vi "6-2_LED VI Curve.vi"() -> ()   [LabVIEW 2014]
doc: "This example demonstrates how to read N channels of analog input from a LINX device.\n------------------------------------\nAuther: Koji Ohashi\nCopyright (c) 2020 Japan LabVIEW Users Group, Volunteer members.\nThis VI is released under the MIT License.\nhttp://opensource.org/licenses/mit-license.php\n------------------------------------"
uses:
  <vilib>/MakerHub/LINX/LMH-LINX.lvlib
  <vilib>/MakerHub/LINX/Public/Peripherals/Analog/Analog Read N Chans.vi
  <vilib>/MakerHub/LINX/Public/Utilities/Open Serial.vi
panel:
  in  "Add Data":bool
  in  "regression analysis":bool
  in  "Resistor (ƒ¶)":dbl=100.0 format="%#_13g"
  out "LED VI characteristics":cluster{dbl[], dbl[]}[](graph)
  in  "AI Channel(s)":u8[](array[numeric])=[0, 1, 2]
  in  "Stop Button":bool
  out "Analog Data":T1(graph)
  in  "Serial Port":refnum<visa-resource-name>
  # "LINX Device Settings"
  # "Model formula used for regression analysis"
  # "n: Ideal diode factor\nI0: Reverse saturation current\ne: Napier number\nr: Internal resistance"
  # "e: elementary charge\nk: Boltzmann constant\nT: Absolute temperature"
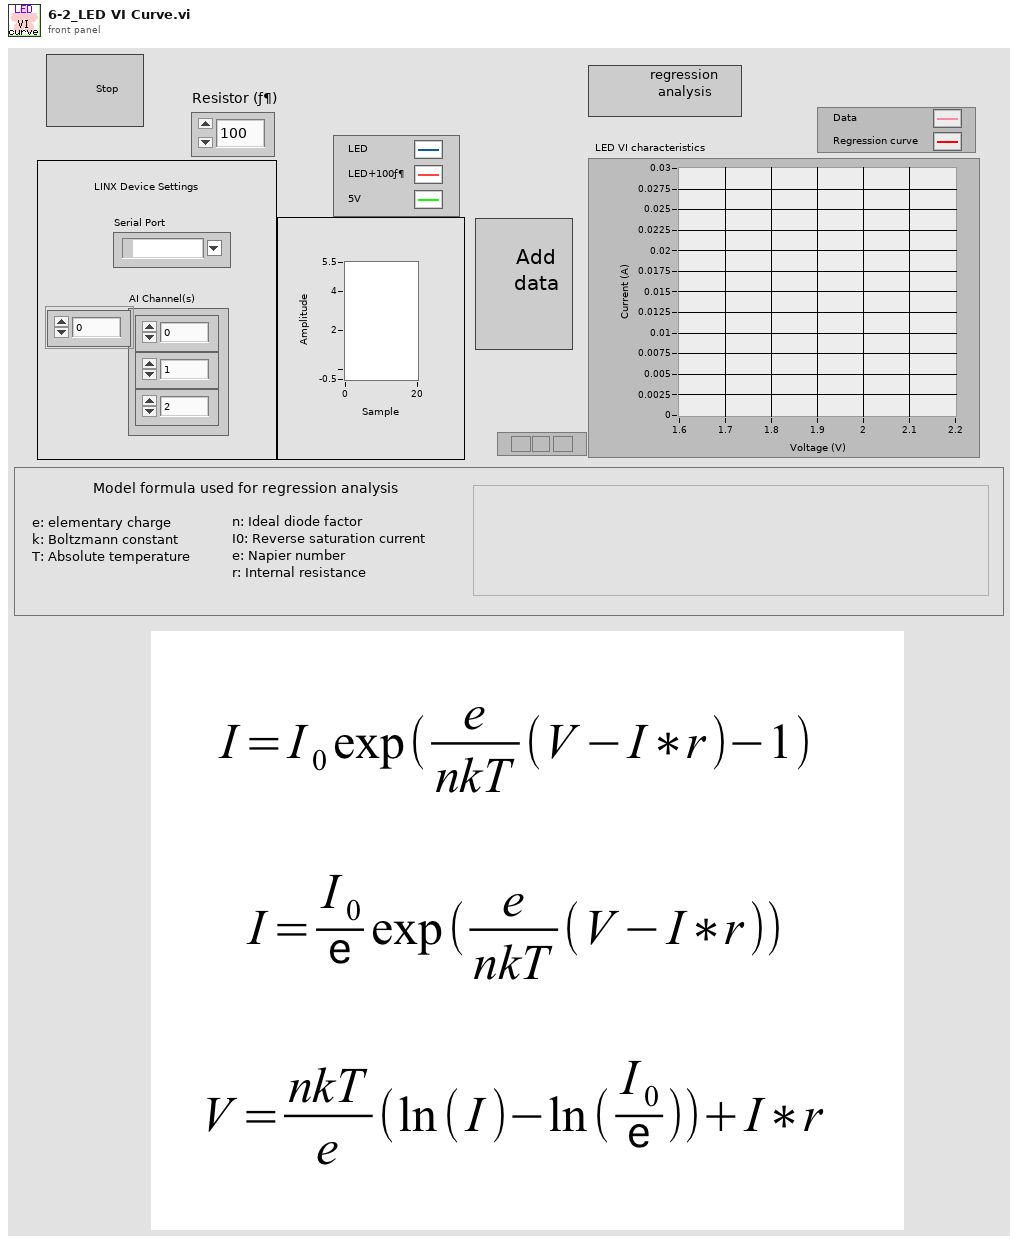
[diagram p1: front panel]
types:
  T1 = cluster{"Voltages[0]":dbl, "Voltages[1]":dbl, "Voltages[2]":dbl}
  T2 = typedef "LMH-LINX.lvlib/LINX Ref.ctl" = cluster{"IO":T3, "Interface":T4, "LINX Device Config":T5}
  T3 = typedef "LMH-LINX.lvlib/Platform.ctl" = enum16{"Remote", "Local"}
  T4 = typedef "LMH-LINX.lvlib/Interface.ctl" = enum16{"Serial", "TCP"}
  T5 = typedef "LMH-LINX.lvlib/Device.lvlib/LINX Device Config.ctl" = cluster{"Interface":T4, "COM Port":refnum<visa-resource-name>, "TCP Configuration":T6, "Device Family":u8, "Device ID":u8, "Device Name":string, "TCP Ref":refnum<k5>, "Channels":T7}
  T6 = typedef "LMH-LINX.lvlib/Device.lvlib/TCP Config.ctl" = cluster{"IP Address":string, "Port":u16}
  T7 = typedef "LMH-LINX.lvlib/Channels.ctl" = cluster{"DI":u8[], "DO":u8[], "AI":u8[], "AO":u8[], "PWM":u8[], "QE":u8[], "UART":u8[], "I2C 2":u8[], "SPI":u8[], "CAN":u8[], "Servo":u8[], "AI Ref (V)":dbl, "AI Resolution (Bits)":u8, "AO Ref (V)":dbl, "AO Resolution (Bits)":u8}
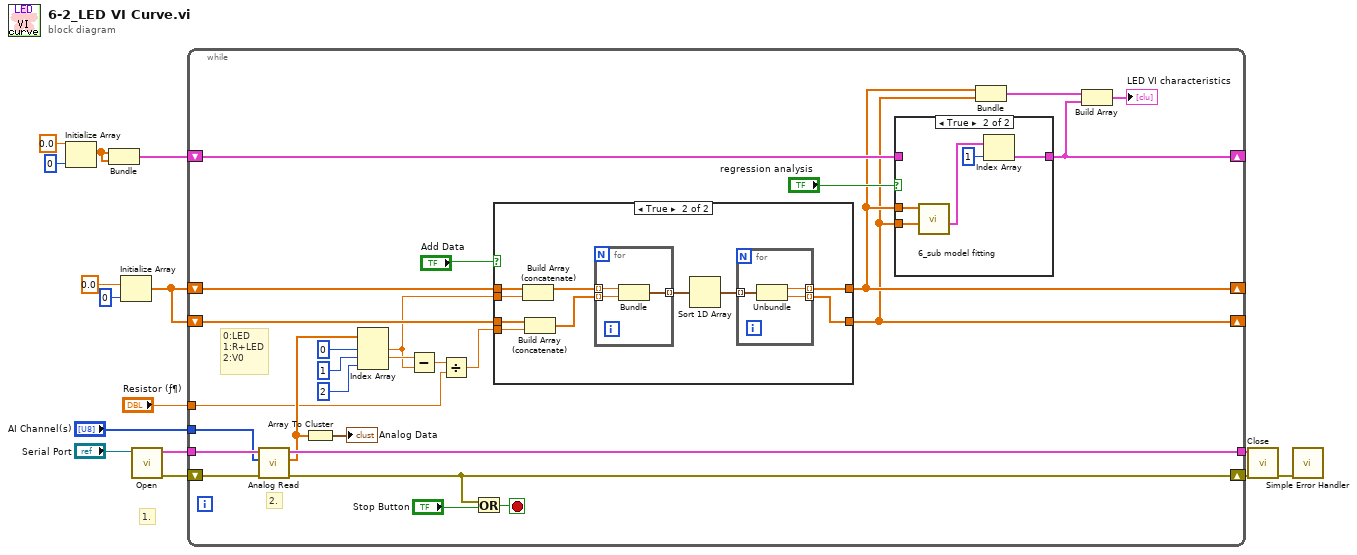
[diagram p0: block diagram]
diagram:
  # "1."
  n1 = Initialize Array(0.0 ("element"), 0 ("dimension size")) -> (w2:dbl[])
  n2 = Bundle(w2, w2) -> (w1:cluster{dbl[], dbl[]})  [unwired: 1 in]
  n3 = Initialize Array(0.0 ("element"), 0 ("dimension size")) -> (w6:dbl[])
  n4 = call-poly <vilib>:"Open.vi"("Serial Port"="Serial Port") -> ("Error Out"=w14:errorcluster, "LINX Resource"=w15:T2)  [unwired: 8 in, 1 out]
  n5 = while {
    tunnel: w15 -> [w42]
    tunnel: [w40] -> w13
    shift-right: [w37] -> w12
    shift-left: w14 -> [w41]
    tunnel: "AI Channel(s)" -> [w36]
    shift-right: [w21] -> _
    shift-left: w6 -> [w28]
    shift-right: [w20] -> _
    shift-left: w6 -> [w27]
    tunnel: "Resistor (ƒ¶)" -> [w24]
    shift-right: [w18] -> _
    shift-left: w1 -> [w22]
    stop <- w39 stop-if-true
    # "0:LED\n1:R+LED\n2:V0"
    # "2."
    n6 = call-poly <vilib>:"Analog Read.vi"("Error In"=w41, "AI Channel(s)"=w36, "LINX Resource"=w42) -> ("Error Out"=w37:errorcluster, "Voltages"=w34:dbl[], "LINX Resource"=w40:T2)  [unwired: 5 in, 1 out]
    n7 = Array To Cluster(array=w34) -> (cluster=→"Analog Data":T1)
    n8 = Index Array(array=w34, index #1=0 ("index"), index #2=1 ("index"), index #3=2 ("index")) -> (element #1=w26:dbl, element #2=w30:dbl)  [unwired: 1 out]
    n9 = Subtract(x=w30, y=w26) -> (x-y=w29:dbl)
    n10 = Divide(x=w29, y=w24) -> (x/y=w25:dbl)
    n11 = Or(x=w37, y="Stop Button") -> (x .or. y?=w39:bool)
    n12 = case shown="TRUE" "Add Data" {
      tunnel: w28 -> [w50 w60]
      tunnel: w27 -> [w49 w58]
      tunnel: [w50 w53] -> w21
      tunnel: [w49 w51] -> w20
      tunnel: w26 -> [_ w59]
      tunnel: w25 -> [_ w57]
      frame False {
      }
      frame True {
        n13 = Build Array (concatenate)(w60, w59) -> (w54:dbl[])
        n14 = Build Array (concatenate)(w58, w57) -> (w52:dbl[])
        n15 = for {
          tunnel: w54 -> [w66] mode=indexing
          tunnel: w52 -> [w65] mode=indexing
          tunnel: [w64] -> w55 mode=indexing
          n16 = Bundle("Numeric Control"=w66, "element"=w65) -> (w64:cluster{"Numeric Control":dbl, "element":dbl})  [unwired: 1 in]
        }
        n17 = Sort 1D Array(array=w55) -> (sorted array=w56:cluster{"Numeric Control":dbl, "element":dbl}[])
        n18 = for {
          tunnel: w56 -> [w63] mode=indexing
          tunnel: [w62] -> w53 mode=indexing
          tunnel: [w61] -> w51 mode=indexing
          n19 = Unbundle(w63) -> ("Numeric Control"=w62:dbl, "element"=w61:dbl)
        }
      }
    }
    n20 = case shown="TRUE" "regression analysis" {
      tunnel: w21 -> [_ w48]
      tunnel: w20 -> [_ w47]
      tunnel: w22 -> [w43 _]
      tunnel: [w43 w44] -> w18
      frame False {
      }
      frame True {
        n21 = call "6_sub model fitting.vi"("LED I data"=w47, "LED V data"=w48) -> ("LED VI characteristics (regression considering internal resistance)"=w46:cluster{dbl[], dbl[]}[])  [unwired: 7 in, 2 out]
        n22 = Index Array(array=w46, index=1) -> (element=w44:cluster{dbl[], dbl[]})
      }
    }
    n23 = Bundle(w21, w20) -> (w19:cluster{dbl[], dbl[]})  [unwired: 1 in]
    n24 = Build Array(w19, w18) -> (→"LED VI characteristics":cluster{dbl[], dbl[]}[])
  }
  n25 = call <vilib>:"Close.vi"("Error In"=w12, "LINX Resource"=w13) -> ("Error Out"=w10:errorcluster)  [unwired: 9 in]
  n26 = call <vilib>:"Simple Error Handler.vi"("error in (no error)"=w10) -> ()  [unwired: 4 in, 5 out]
